vi "findCircleVelocity.vi"(0 "Game in":refnum<class "Game.lvclass">, 5 "theta":dbl format="%#_13g", 7 "v_backtracking":dbl format="%#_13g", 11 "error in (no error)":errorcluster, 12 "v_ang":dbl format="%#_13g", 13 "L_limit":dbl format="%#_13g") -> (4 "Game out":refnum<class "Game.lvclass">, 6 "L":dbl, 8 "v_circle":dbl, 15 "error out":errorcluster)   [LabVIEW 2020, in "Game.lvclass"]
uses:
  Game.lvclass
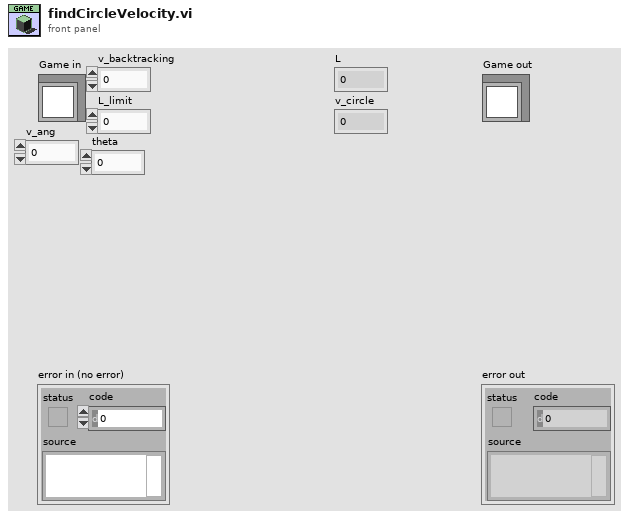
[diagram p1: front panel]
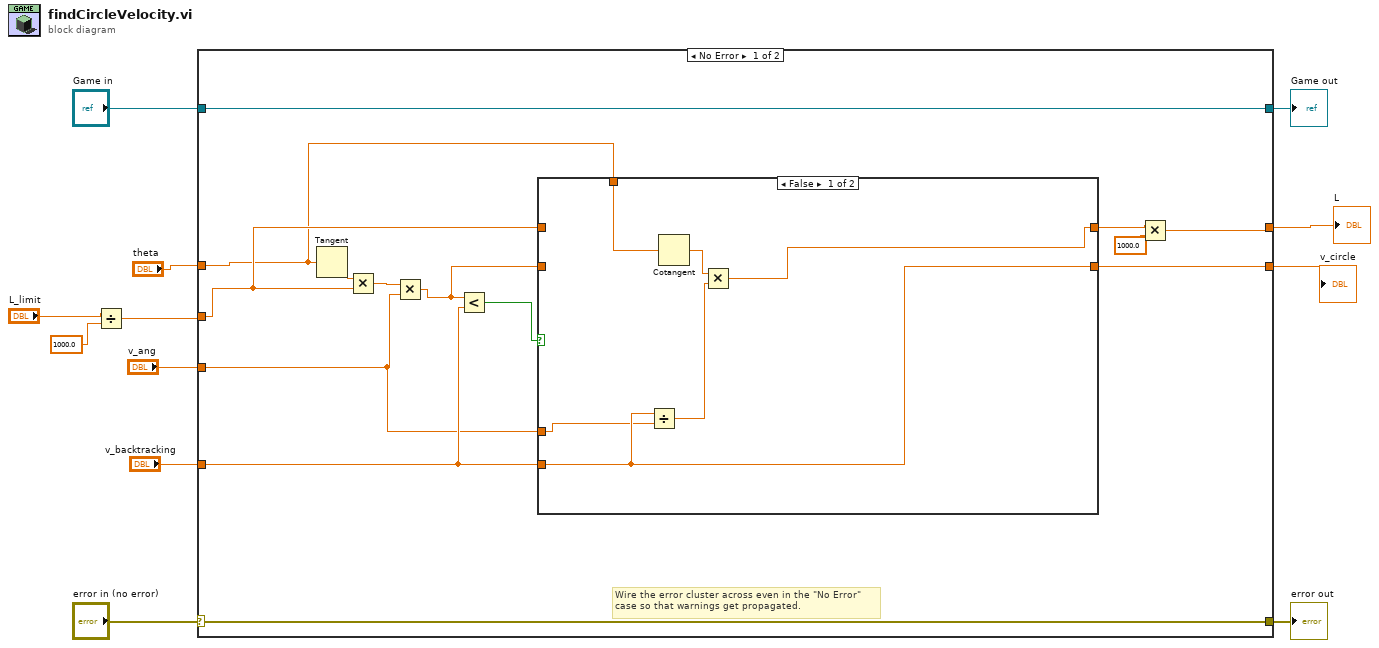
[diagram p0: block diagram]
diagram:
  n1 = Divide(x="L_limit", y=1000.0) -> (x/y=w1:dbl)
  n2 = case shown="No Error" "error in (no error)" {
    selector: "error in (no error)" -> [w25 w36]
    tunnel: [w25 w36] -> w11
    tunnel: [w26 w35] -> w9
    tunnel: "Game in" -> [w26 w35]
    tunnel: w1 -> [w14 _]
    tunnel: "theta" -> [w13 _]
    tunnel: "v_ang" -> [w19 _]
    tunnel: "v_backtracking" -> [w22 _]
    tunnel: [w15 _] -> w5
    tunnel: [w18 _] -> w4
    frame No Error {
      # "Wire the error cluster across even in the \"No Error\"\ncase so that warnings get propagated."
      n3 = Tangent(1:w13) -> (0:w24:dbl)
      n4 = Multiply(x=w24, y=w14) -> (x*y=w20:dbl)
      n5 = Multiply(x=w20, y=w19) -> (x*y=w21:dbl)
      n6 = Less?(x=w21, y=w22) -> (x < y?=w23:bool)
      n7 = case shown="False" w23 {
        tunnel: w22 -> [w32 _]
        tunnel: w21 -> [_ w34]
        tunnel: [w32 w34] -> w18
        tunnel: w14 -> [_ w33]
        tunnel: [w27 w33] -> w17
        tunnel: w19 -> [w31 _]
        tunnel: w13 -> [w30 _]
        frame False {
          n8 = Divide(x=w32, y=w31) -> (x/y=w28:dbl)
          n9 = Cotangent(1:w30) -> (0:w29:dbl)
          n10 = Multiply(x=w29, y=w28) -> (x*y=w27:dbl)
        }
        frame True {
        }
      }
      n11 = Multiply(x=w17, y=1000.0) -> (x*y=w15:dbl)
    }
    frame Error {
    }
  }
  "error out" <- w11
  "Game out" <- w9
  "L" <- w5
  "v_circle" <- w4
